vi "Esophageal_FastHRME_CameraInitialize.vi"(8 "error in (no error)":errorcluster) -> (0 "error out":errorcluster, 2 "HRME Image Reference":T2, 3 "OMS Camera Reference Out":T1 caption="FastHRME Camera Session Out")   [LabVIEW 2021]
uses:
  <vilib>/userDefined/High Color/IMAQdx.ctl
  <vilib>/vision/Image Controls.llb/IMAQ Image.ctl
  <vilib>/vision/driver/IMAQdx.llb/IMAQdx Acquisition Mode.ctl
  <vilib>/vision/driver/NI_Vision_Acquisition_Software.lvlib
  <resource>/objmgr/imaqdx.rc
panel:
  in  "FastHRME Camera Session":T1="cam2"
  # "SubVI Inputs"
  # "SubVI Outputs"
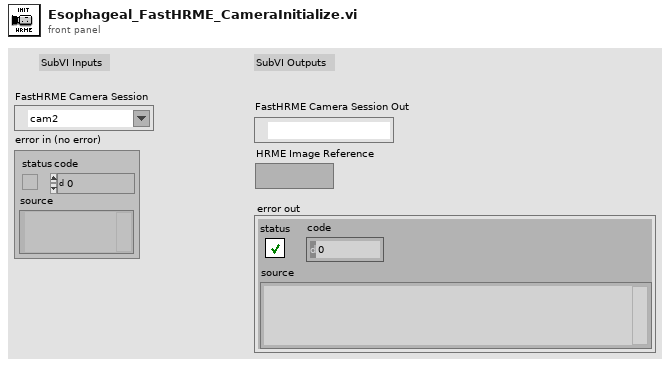
[diagram p1: front panel]
types:
  T1 = typedef "IMAQdx.ctl" = refnum<k21>
  T2 = typedef "IMAQ Image.ctl" = refnum<image>
  T3 = typedef "NI_Vision_Acquisition_Software.lvlib/IMAQdx Acquisition Mode.ctl" = enum32{"One Shot", "Continuous"}
  T4 = typedef "Image Type" = u32
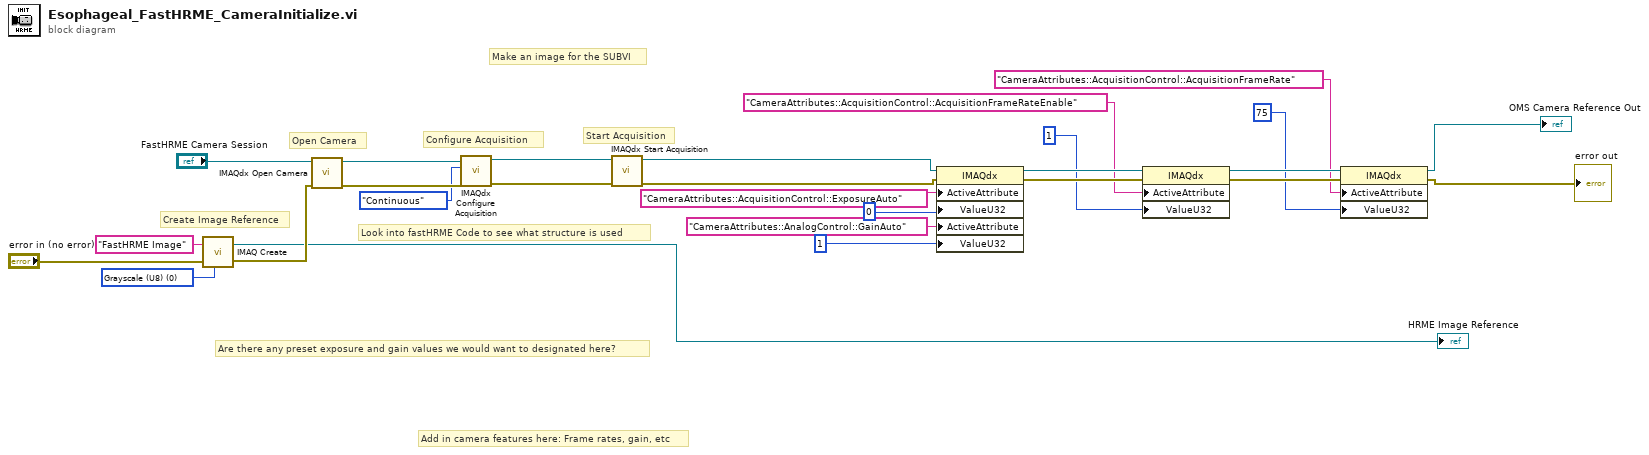
[diagram p0: block diagram]
diagram:
  w26 = T4 0 items=["Grayscale (U8)", "Grayscale (I16)", "Grayscale (SGL)", "Complex (CSG)", "RGB (U32)", "HSL (U32)", "RGB (U64)", "Grayscale (U16)"] ("Image Type")
  # "Add in camera features here: Frame rates, gain, etc"
  # "Are there any preset exposure and gain values we would want to designated here?"
  # "Make an image for the SUBVI"
  # "Start Acquisition"
  # "Look into fastHRME Code to see what structure is used"
  # "Configure Acquisition"
  # "Open Camera"
  # "Create Image Reference"
  n1 = call "IMAQ Create"("Image Name"="FastHRME Image", "Image Type"=w26, "error in (no error)"="error in (no error)") -> ("New Image"=→"HRME Image Reference":T2, "error out"=w19:errorcluster)  [unwired: 2 in]
  n2 = call <vilib>:"IMAQdx Open Camera.vi"("error in"=w19, "Session In"="FastHRME Camera Session") -> ("error out"=w23:errorcluster, "Session Out"=w24:T1)  [unwired: 8 in]
  n3 = call <vilib>:"IMAQdx Configure Acquisition.vi"("error in"=w23, "Continuous?"=IMAQdx_Acquisition_Mode."Continuous", "Session In"=w24) -> ("error out"=w20:errorcluster, "Session Out"=w21:T1)  [unwired: 7 in]
  n4 = call <vilib>:"IMAQdx Start Acquisition.vi"("error in"=w20, "Session In"=w21) -> ("error out"=w12:errorcluster, "Session Out"=w11:T1)  [unwired: 8 in]
  n5 = property class="IMAQdx"(reference=w11, error in=w12, "ActiveAttribute"="CameraAttributes::AcquisitionControl::ExposureAuto", "ValueU32"=u32 0, "ActiveAttribute"="CameraAttributes::AnalogControl::GainAuto", "ValueU32"=u32 1) -> (reference out=w10:T1, error out=w9:errorcluster)
  n6 = property class="IMAQdx"(reference=w10, error in=w9, "ActiveAttribute"="CameraAttributes::AcquisitionControl::AcquisitionFrameRateEnable", "ValueU32"=u32 1) -> (reference out=w6:T1, error out=w5:errorcluster)
  n7 = property class="IMAQdx"(reference=w6, error in=w5, "ActiveAttribute"="CameraAttributes::AcquisitionControl::AcquisitionFrameRate", "ValueU32"=u32 75) -> (reference out=→"OMS Camera Reference Out":T1, error out=→"error out":errorcluster)
